vi "Day 1 task 2.vi"() -> ()   [LabVIEW 2022 SP3]
uses:
  <vilib>/regexp/Match Regular Expression.xnode
panel:
  out "spreadsheet string 2":string
  out "spreadsheet string":string
  out "sum":i64
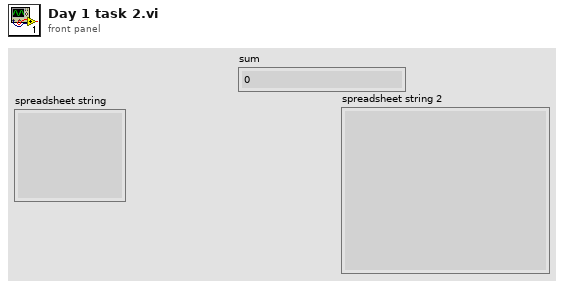
[diagram p1: front panel]
diagram:
  (unwired) "xfgqc36oneightvlx"
  (unwired) "two1nine\neightwothree\nabcone2threexyz\nxtwone3four\n4nineeightseven2\nzoneight234\n7pqrstsixteen"
  # "Should be 38!"
  n1 = Spreadsheet String To Array(delimiter (Tab)="\n", format string="%s", spreadsheet string="cmpptgjc3qhcjxcbcqgqkxhrms\n9sixonefour\neighttwo2twofour9\n7eightseveneightthree\ntlnllks2jcfdlgsjbhpfnineone\none44fivesevenjzsfzddg\n787seveneight75five\n7q7nine3\nhlqphphn5dtzzbqvk3three8seven\nninekkbvsfq8seven7321bpdcdh\n9kxgfxntgdzs1ns5\nnineblxtnrt79t8fourbcqdzpb\n3mjqgthreeseven36gkvvvqppx\nzpcvkjjqeight94one82mrvfzdvlgjgkhj\nnine11\nrnscpccv8\n7eightrcqnbtkn\nfour31zqgrccc4eight\ntwo65fourfourt1\ntwomg2764threesix\n546grjcrsix9\n4ffourfourff1\ndpfkcrzjxr8four\n641one\nkseven8\ntwo4four\nldzpzgch325hsttqvmp9foureightmvsknbd\nonexrbclqlnvp5kqtrsgdh8nine\nrk9qfzvszksjqsixg\ndcnhlcqzhthreebhrnfgjbfive1threetwo53\n1tw...", array type (2D Dbl)=string[] []) -> (array=w13:string[])
  n2 = for {
    tunnel: w13 -> [w29] mode=indexing
    tunnel: string[] ["zero", "one", "two", "three", "four", "five", "six", "seven", "eight", "nine"] -> [w27]
    tunnel: [w25] -> w11 mode=indexing
    tunnel: [w19] -> w9 mode=indexing
    tunnel: [w18] -> w7 mode=indexing
    n3 = while {
      tunnel: "\\d|one|two|three|four|five|six|seven|eight|nine" ("regular expression") -> [w43]
      tunnel: w27 -> [w42]
      tunnel: [w39] -> w19 mode=indexing if=w36
      tunnel: w29 -> [w44]
      shift-right: [w32] -> _
      shift-left: 0 -> [w35]
      stop <- w36 continue-if-true
      n4 = xnode "Match Regular Expression"("input string"=w44, "regular expression"=w43, "offset (0)"=w35) -> ("whole match"=w33:string, "offset past match"=w34:i32)  [unwired: 3 in, 3 out]
      n5 = String Length(string=w33) -> (length=w31:i32)
      n6 = Decrement(x=w31) -> (x-1=w30:i32)
      n7 = Subtract(x=w34, y=w30) -> (x-y=w32:i32)
      n8 = Greater Or Equal To 0?(x=w34) -> (x >= 0?=w36:bool)
      n9 = Search 1D Array(1D array=w42, element=w33) -> (index of element=w38:i32)  [unwired: 1 in]
      n10 = Not Equal?(x=w38, y=-1) -> (x != y?=w40:bool)
      n11 = Number To Decimal String(number=w38) -> (decimal integer string=w37:string)  [unwired: 1 in]
      n12 = Select(t=w37, s=w40, f=w33) -> (s? t:f=w39:string)
    }
    n13 = Delete From Array(array=w19) -> (deleted portion=w22:string, array with subset deleted=w26:string[])  [unwired: 2 in]
    n14 = Index Array(array=w26) -> (element=w21:string)  [unwired: 1 in]
    n15 = Empty String/Path?(string/path=w21) -> (empty?=w23:bool)
    n16 = Select(t=w22, s=w23, f=w21) -> (s? t:f=w20:string)
    n17 = Concatenate Strings(w20, w22) -> (w18:string)
    n18 = Decimal String To Number(string=w18, default (0L)=i64 0 ("default (0 I32)")) -> (number=w25:i64)  [unwired: 1 in, 1 out]
  }
  n19 = Add Array Elements(numeric array=w11) -> (sum=→"sum":i64)
  n20 = call <vilib>:"Space Constant.vi"() -> ("String"=w3:string)
  n21 = Array To Spreadsheet String(delimiter (Tab)=w3, array=w9, 3:"%s" ("format string")) -> (spreadsheet string=→"spreadsheet string":string)
  n22 = Array To Spreadsheet String(delimiter (Tab)="\n", array=w7, 3:"%s" ("format string")) -> (spreadsheet string=→"spreadsheet string 2":string)
